vi "Material-Line3-Aquisition.vi"(8 "error in (no error)":errorcluster, 11 "Material-RunTest in":refnum<class "Material-RunTest.lvclass">) -> (0 "error out":errorcluster, 3 "Material-RunTest out":refnum<class "Material-RunTest.lvclass">)   [LabVIEW 2013, in "Material-RunTest.lvclass"]
uses:
  Material-RunTest.lvclass
  Material-RunTest.lvclass/Material-RunTest.ctl
  <instrlib>/Keyence LK-G5000/Public/enum/LKIF_OUTNO.ctl
  <instrlib>/Keyence LK-G5000/Keyence LK-G5000.lvlib
  Motion Control/Motion-ControlAll.lvclass
panel:
  out "Laser Value":sgl format="%_6g"
  out "Init Meas1":dbl[](array[numeric])
  out "stop collecting":bool
  out "Meas 1 Dyn Data":dbl[](graph)
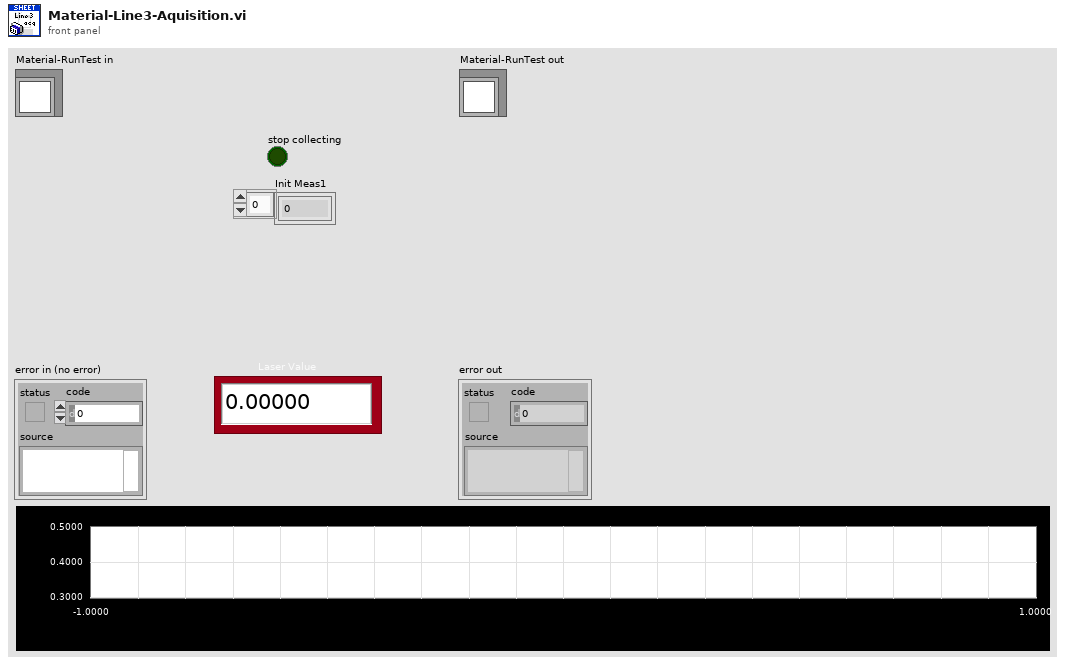
[diagram p1: front panel]
types:
  T1 = typedef "Keyence LK-G5000.lvlib/LKIF_OUTNO.ctl" = i32
  T2 = typedef "Keyence LK-G5000.lvlib/LKIF_FLOATRESULT.ctl" = i32
  T3 = cluster{"OutNo":i32, "LKIF_FLOATRESULT":T2, "Value":sgl}[]
  T4 = cluster{"OutNo":i32, "LKIF_FLOATRESULT":T2, "Value":sgl}
  T5 = cluster{waveform(dbl), waveform(dbl), waveform(dbl)}
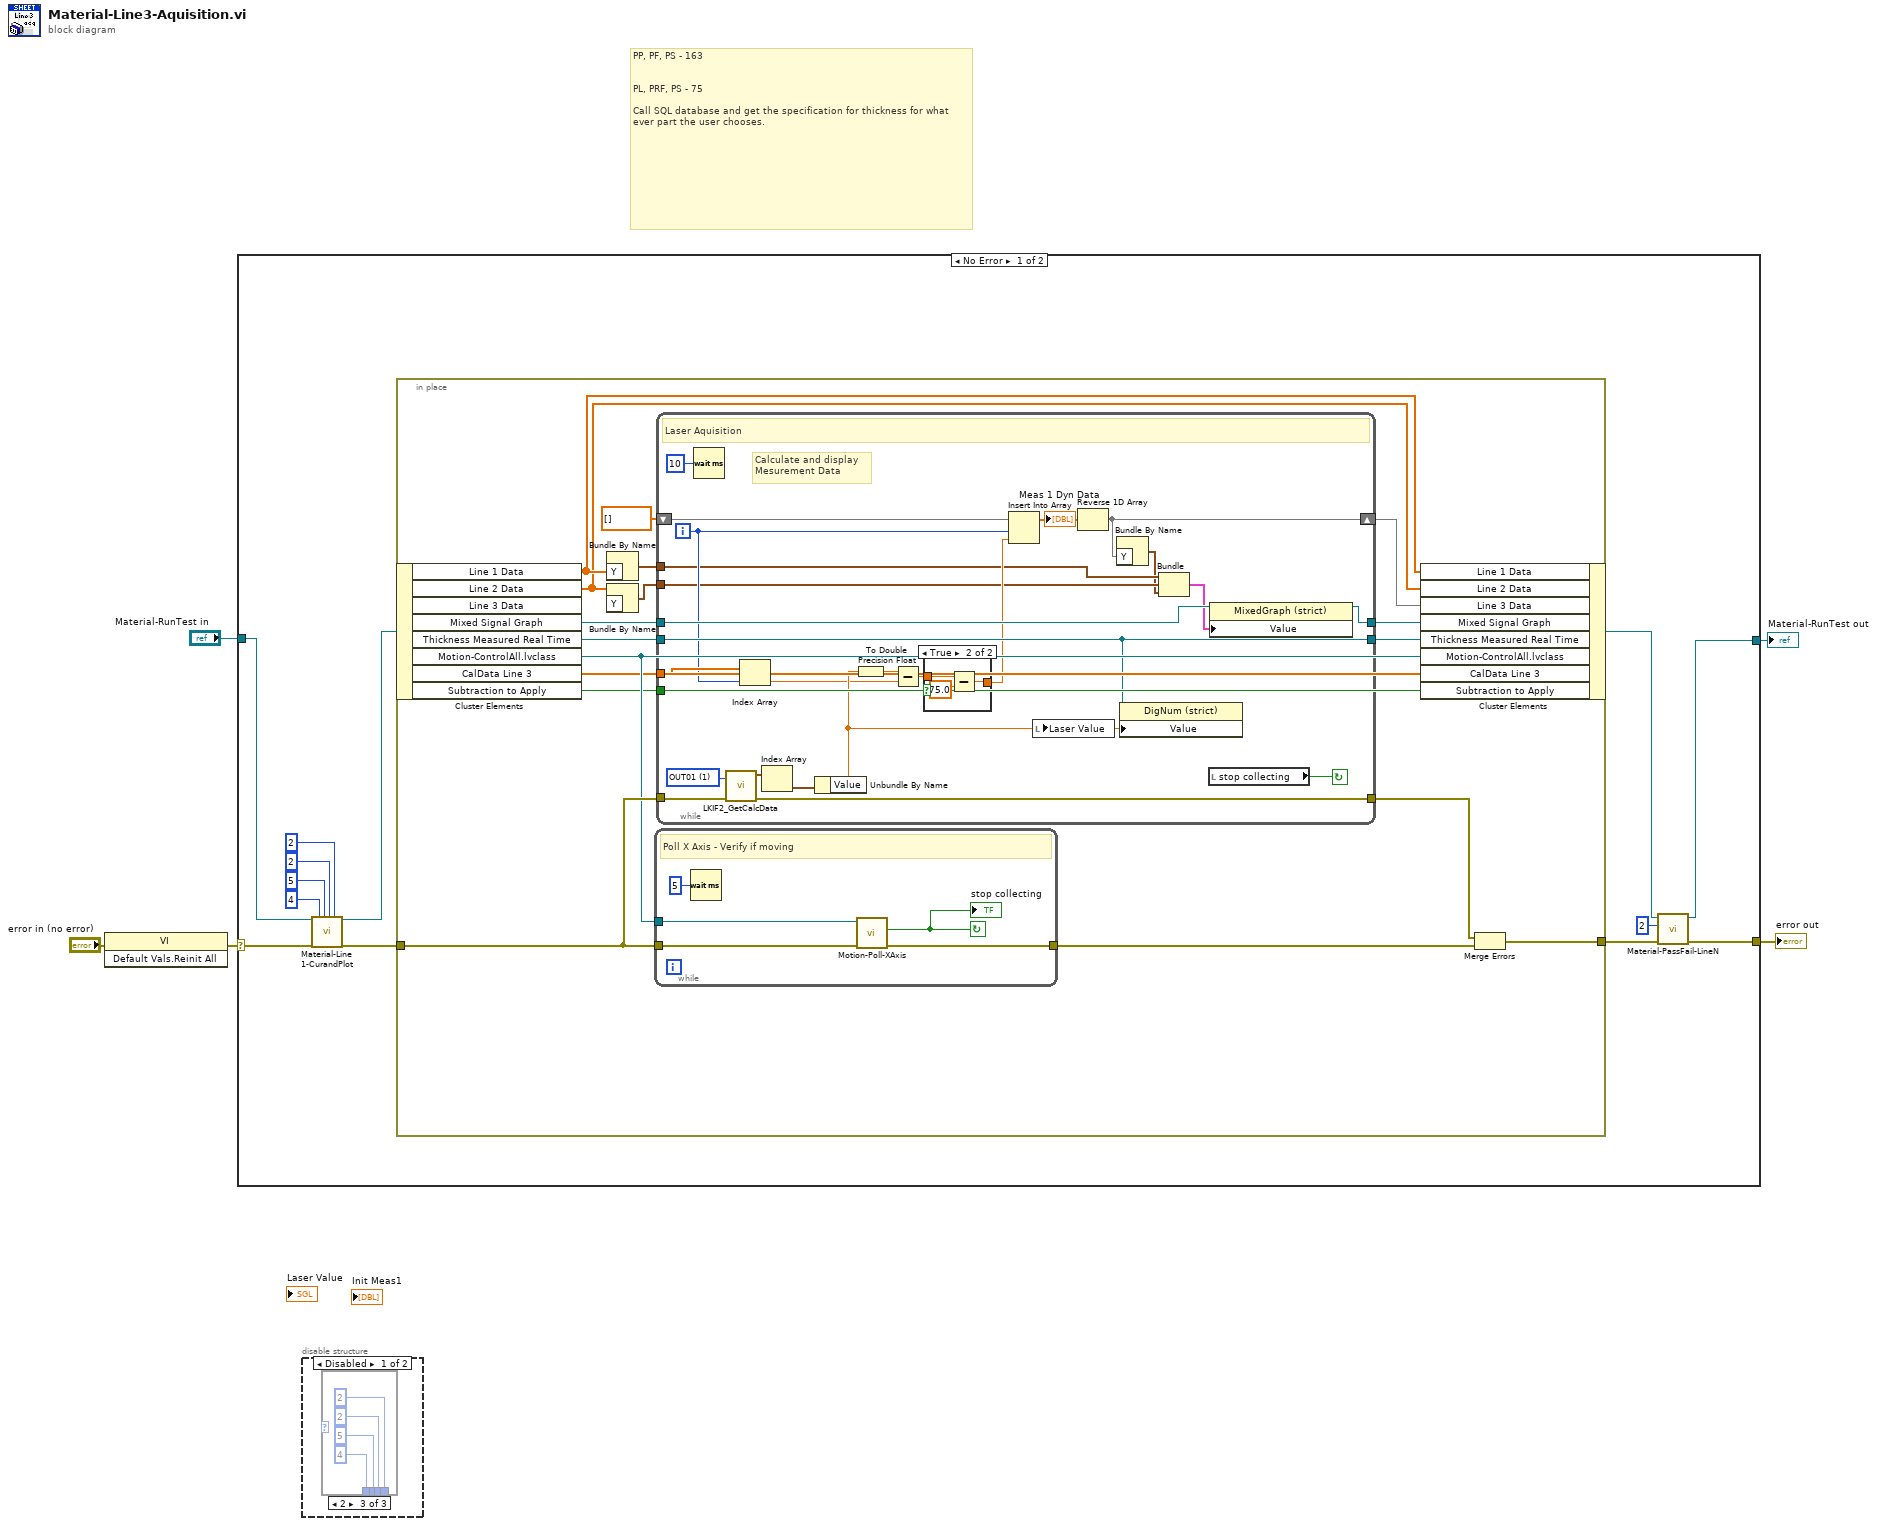
[diagram p0: block diagram]
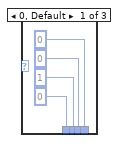
[diagram p2: hidden frame]
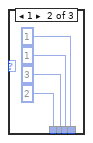
[diagram p3: hidden frame]
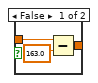
[diagram p5: hidden frame]
diagram:
  # "PP, PF, PS - 163\n\n\nPL, PRF, PS - 75\n\nCall SQL database and get the specification for thickness for what ever part the user chooses."
  n1 = invoke class="VI" method="Default Vals.Reinit All"(error in="error in (no error)") -> (error out=w1:errorcluster)  [unwired: 2 in, 2 out]
  n2 = case shown="No Error" w1 {
    selector: w1 -> [w17 w73]
    tunnel: [w10 w73] -> w5
    tunnel: [w11 w72] -> w3
    tunnel: "Material-RunTest in" -> [w18 w72]
    frame No Error {
      n3 = call "Material-Line 1-CurandPlot.vi"("Material-RunTest in"=w18, "error in (no error)"=w17, "Active Cursor Max"=u32 4, "Active Cursor Min"=u32 5, "Active Y Scale"=2, "Active Plot"=u32 2) -> ("Material-RunTest out"=w15:refnum<class "Material-RunTest.lvclass">, "error out"=w16:errorcluster)  [unwired: 12 in]
      n4 = in-place {
        in-place-border: w16 -> [w35]
        in-place-border: [w26] -> w14
        n5 = in-place-cluster #1(w15) -> ("Line 1 Data"=w20:dbl[], "Line 2 Data"=w19:dbl[], "Mixed Signal Graph"=w32:refnum<vi>, "Thickness Measured Real Time"=w34:refnum<vi>, "Motion-ControlAll.lvclass"=w29:refnum<class "Motion-ControlAll.lvclass">, "CalData Line 3"=w24:dbl[], "Subtraction to Apply"=w23:bool)  [unwired: 1 out]
        n6 = Bundle By Name("Y"=w20) -> (w22:waveform(dbl))  [unwired: 1 in]
        n7 = Bundle By Name("Y"=w19) -> (w21:waveform(dbl))  [unwired: 1 in]
        n8 = while {
          tunnel: w35 -> [w39]
          tunnel: [w37] -> w28
          tunnel: w29 -> [w38]
          stop <- w36 continue-if-true
          # "Poll X Axis - Verify if moving"
          n9 = Wait (ms)(milliseconds to wait=u32 5) -> ()  [unwired: 1 out]
          n10 = call "Motion-Poll-XAxis.vi"("error in (no error)"=w39, "Motion-ControlAll in"=w38) -> ("error out"=w37:errorcluster, "X axis \nstopped"=w36:bool)  [unwired: 7 in, 1 out]
          "stop collecting" <- w36
        }
        n11 = while {
          tunnel: w35 -> [w65]
          tunnel: [w61] -> w27
          tunnel: w34 -> [w51]
          shift-right: [w53] -> w25
          shift-left: dbl[] [] -> [w58]
          tunnel: w32 -> [w55]
          tunnel: [w52] -> w31
          tunnel: [w51] -> w30
          tunnel: w24 -> [w50]
          tunnel: w23 -> [w46]
          tunnel: w22 -> [w43]
          tunnel: w21 -> [w42]
          i -> [w49]
          stop <- w59 continue-if-true
          w64 = T1 1 items=["OUT01"=1, "OUT02"=2, "OUT03"=4, "OUT04"=8, "OUT05"=16, "OUT06"=32, "OUT07"=64, "OUT08"=128, "OUT09"=256, "OUT10"=512, "OUT11"=1024, "OUT12"=2048, "ALL OUT"=4095] ("OutNo (OUT1)")
          # "Calculate and display \nMesurement Data"
          # "Laser Aquisition"
          n12 = Wait (ms)(milliseconds to wait=u32 10) -> ()  [unwired: 1 out]
          n13 = call <instrlib>:"LKIF2_GetCalcData.vi"("OutNo (OUT1)"=w64, "error in (no error)"=w65) -> ("error out"=w61:errorcluster, "CalcData"=w63:T3)  [unwired: 8 in]
          n14 = Index Array(array=w50, index=w49) -> (element=w47:dbl)
          n15 = Index Array(array=w63) -> (element=w62:T4)  [unwired: 1 in]
          n16 = Unbundle By Name(w62) -> ("Value"=w57:sgl)
          n17 = To Double Precision Float(number=w57) -> (double precision float=w48:dbl)
          n18 = Subtract(x=w48, y=w47) -> (x-y=w45:dbl)
          n19 = case shown="True" w46 {
            tunnel: w45 -> [w67 w71]
            tunnel: [w66 w69] -> w44
            frame False {
              n20 = Subtract(x=w67, y=163.0) -> (x-y=w66:dbl)
            }
            frame True {
              n21 = Subtract(x=w71, y=75.0) -> (x-y=w69:dbl)
            }
          }
          n22 = Insert Into Array(array=w58, index=w49, new element=w44) -> (w56:dbl[])
          "Meas 1 Dyn Data" <- w56
          n23 = local write "Laser Value"(w57) -> ()
          n24 = Reverse 1D Array(array=w56) -> (reversed array=w53:dbl[])
          n25 = Bundle By Name("Y"=w53) -> (w41:waveform(dbl))  [unwired: 1 in]
          n26 = property class="DigNum (strict)"(reference=w51, "Value"=w57) -> ()  [unwired: 1 in, 2 out]
          n27 = Bundle(w43, w42, w41) -> (w54:T5)  [unwired: 1 in]
          n28 = local read "stop collecting"() -> (w59:bool)
          n29 = property class="MixedGraph (strict)"(reference=w55, "Value"=w54) -> (reference out=w52:refnum<vi>)  [unwired: 1 in, 1 out]
        }
        n30 = in-place-cluster #1("Line 1 Data"=w20, "Line 2 Data"=w19, "Line 3 Data"=w25, "Mixed Signal Graph"=w31, "Thickness Measured Real Time"=w30, "Motion-ControlAll.lvclass"=w29, "CalData Line 3"=w24, "Subtraction to Apply"=w23) -> (w13:refnum<class "Material-RunTest.lvclass">)
        n31 = Merge Errors(w27, w28) -> (w26:errorcluster)
      }
      n32 = call "Material-PassFail-LineN.vi"("error in (no error)"=w14, "Line?"=2, "Material-RunTest in"=w13) -> ("error out"=w10:errorcluster, "Material-RunTest out"=w11:refnum<class "Material-RunTest.lvclass">)  [unwired: 7 in]
    }
    frame Error {
    }
  }
  "error out" <- w5
  "Material-RunTest out" <- w3
  n33 = disable-structure shown="Disabled" {
    frame Disabled {
      n34 = case shown="2" {
        selector: _ -> [_ _ _]
        tunnel: [u32 0 ("Active Cursor Max") u32 2 ("Active Cursor Max") u32 4 ("Active Cursor Max")] -> _
        tunnel: [u32 1 ("Active Cursor Min") u32 3 ("Active Cursor Min") u32 5 ("Active Cursor Min")] -> _
        tunnel: [0 ("Active Y Scale") 1 ("Active Y Scale") 2 ("Active Y Scale")] -> _
        tunnel: [u32 0 ("Active Plot") u32 1 ("Active Plot") u32 2 ("Active Plot")] -> _
        frame 0, Default {
        }
        frame 1 {
        }
        frame 2 {
        }
      }
    }
    frame Enabled {
    }
  }
